vi "GetClassProperties.vi"(0 "reference in":refnum<class "ClassWriterGOOP400.lvclass">, 1 "LvClassItem":refnum<vi>, 2 "TreeControl":refnum<vi>, 5 "error in (no error)":errorcluster) -> (14 "reference out":refnum<class "ClassWriterGOOP400.lvclass">, 19 "error out":errorcluster)   [LabVIEW 2014, in "ClassWriterGOOP400.lvclass"]
uses:
  <resource>/Framework/Providers/Open_GDS/ClassProviders/Provider_EndevoGOOP400/ClassWriterGOOP400_class/ClassWriterGOOP400.lvclass
panel:
  out "ClassClasses":string[](array[string])
  out "ObjectClasses":string[](array[string])
  out "ClassAttributes":string[][](array[string])
  out "ObjectAttributes":string[][](array[string])
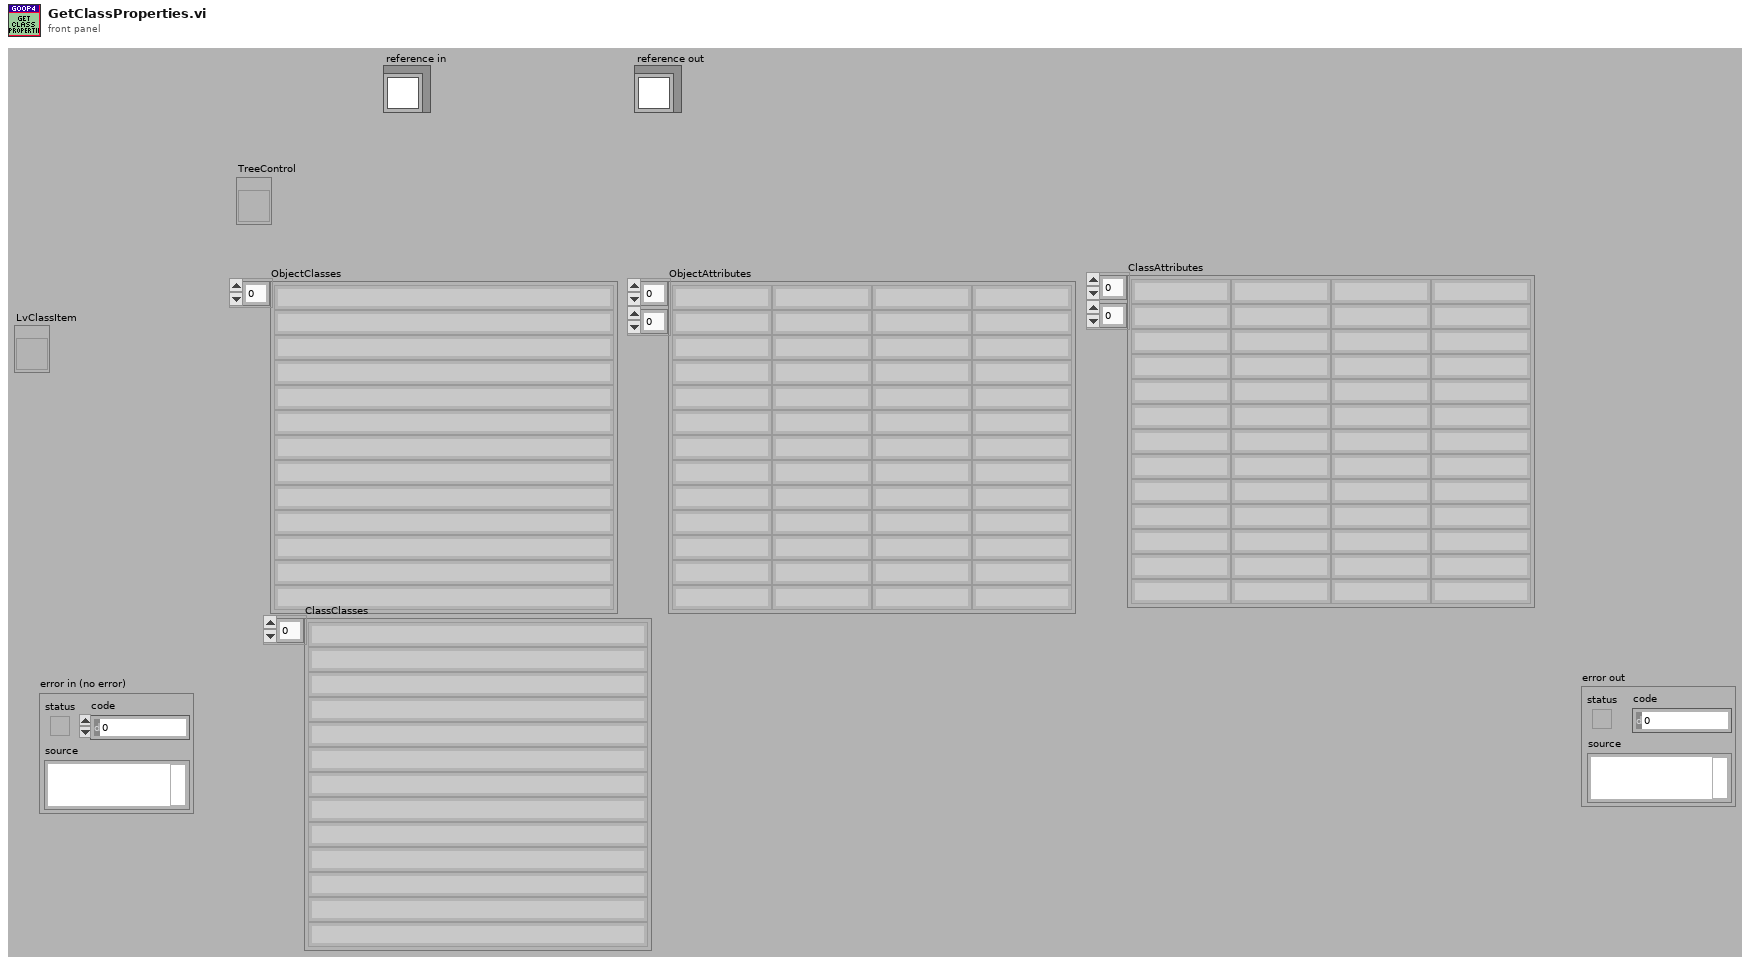
[diagram p1: front panel]
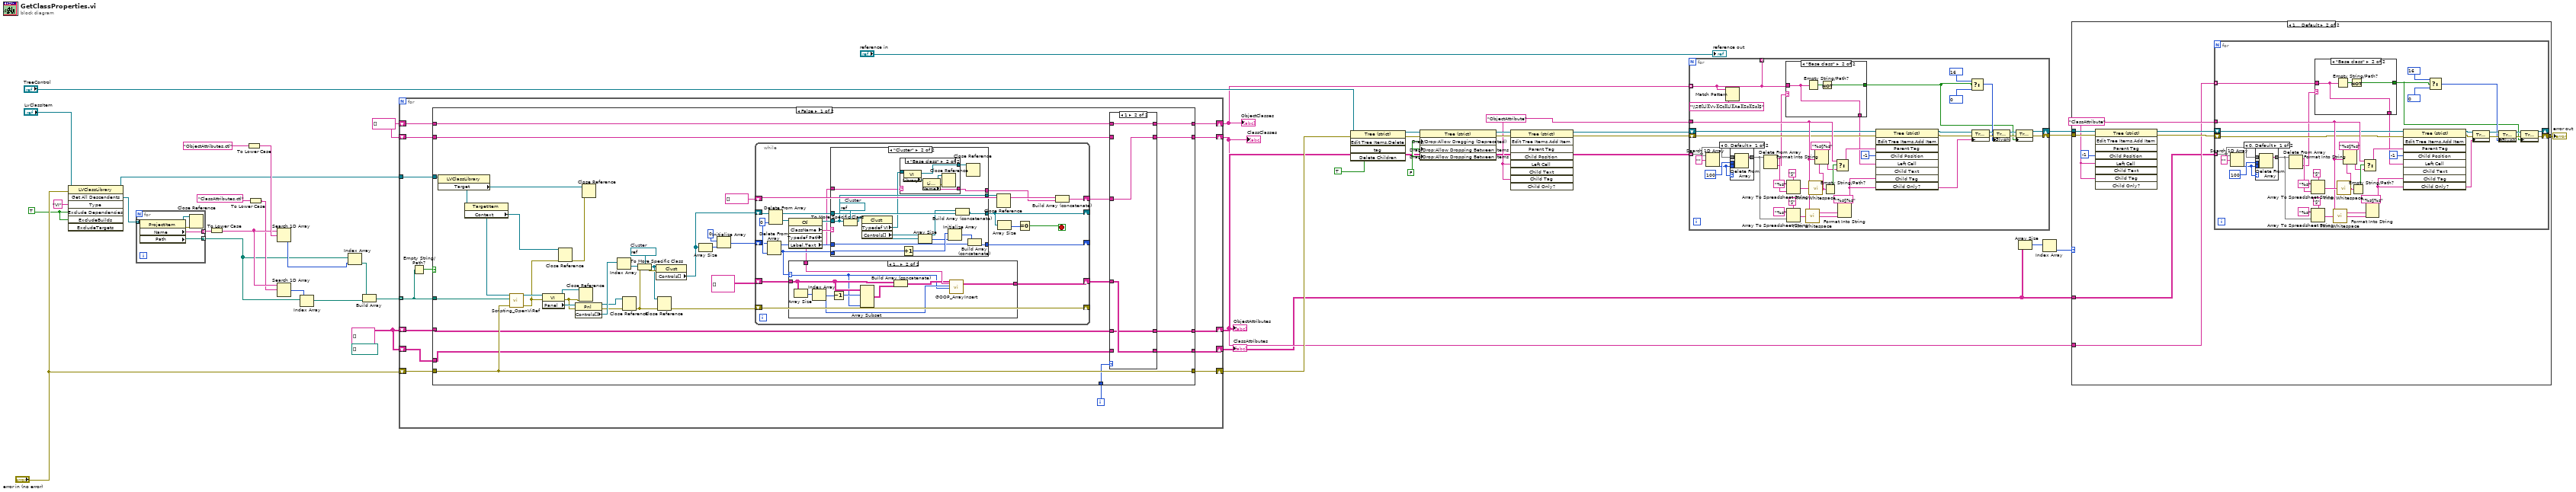
[diagram p0: block diagram]
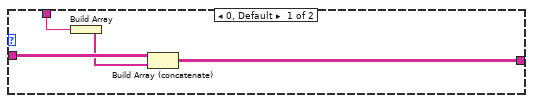
[diagram p8: hidden frame]
diagram:
  w5 = TRUE ("ExcludeDependencies")
  w17 = FALSE ("Drag/Drop:Allow Dragging (Deprecated)")
  w12 = "ObjectAttribute" ("Left Cell String(Main name)")
  w23 = string[] []
  (unwired) path[] []
  w40 = string[][] []
  n1 = invoke class="LVClassLibrary" method="Get All Descendents"(reference="LvClassItem", error in="error in (no error)", "Type"="VI", "Exclude Dependencies"=w5, "ExcludeBuilds"=w5) -> (reference out=w1:refnum<vi>, "All Descendents"=w38:refnum<vi>[])  [unwired: 2 in, 5 out]
  n2 = for {
    tunnel: w38 -> [w46] mode=indexing
    tunnel: [w45] -> w37 mode=indexing
    tunnel: [w44] -> w31 mode=indexing
    n3 = property class="ProjectItem"(reference=w46) -> (reference out=w43:refnum<vi>, error out=w42:errorcluster, "Name"=w45:string, "Path"=w44:path)  [unwired: 1 in]
    n4 = Close Reference(reference=w43, error in (no error)=w42) -> ()  [unwired: 1 out]
  }
  n5 = To Lower Case(string=w37) -> (all lower case string=w35:string[])
  n6 = To Lower Case(string="ObjectAttributes.ctl") -> (all lower case string=w36:string)
  n7 = To Lower Case(string="ClassAttributes.ctl") -> (all lower case string=w34:string)
  n8 = Search 1D Array(1D array=w35, element=w36) -> (index of element=w33:i32)  [unwired: 1 in]
  n9 = Search 1D Array(1D array=w35, element=w34) -> (index of element=w32:i32)  [unwired: 1 in]
  n10 = Index Array(array=w31, index=w32) -> (element=w25:path)
  n11 = Index Array(array=w31, index=w33) -> (element=w26:path)
  n12 = Build Array(w26, w25) -> (w30:path[])
  n13 = for {
    shift-right: [w60] -> w9
    shift-left: "error in (no error)" -> [w59]
    shift-right: [w57] -> w8
    shift-left: w40 -> [w58]
    shift-right: [w55] -> w4
    shift-left: w40 -> [w56]
    tunnel: w30 -> [w54] mode=indexing
    shift-right: [w51] -> w7
    shift-left: w23 -> [w48]
    shift-right: [w50] -> w6
    shift-left: w23 -> [w49]
    tunnel: w1 -> [w47]
    i -> [w52]
    n14 = Empty String/Path?(string/path=w54) -> (empty?=w53:bool)
    n15 = case shown="False" w53 {
      tunnel: [w95 w169] -> w60
      tunnel: w59 -> [w95 w169]
      tunnel: w58 -> [w79 w170]
      tunnel: [w82 w170] -> w57
      tunnel: w56 -> [w81 w168]
      tunnel: [w80 w168] -> w55
      tunnel: w54 -> [w97 _]
      tunnel: w52 -> [w84 _]
      tunnel: [w70 w167] -> w51
      tunnel: [w68 w166] -> w50
      tunnel: w49 -> [w67 w166]
      tunnel: w48 -> [w66 w167]
      tunnel: w47 -> [w64 _]
      frame False {
        w88 = refnum<vi> refnum  # Cluster
        n16 = property class="LVClassLibrary"(reference=w64) -> ("Target"=w65:refnum<vi>)  [unwired: 1 in, 2 out]
        n17 = property class="TargetItem"(reference=w65) -> ("Context"=w61:refnum<vi>)  [unwired: 1 in, 2 out]
        n18 = call <resource>:"Scripting_OpenViRef.vi"("error in"=w95, "ViPath/ViName/Viref"=w97, "AppRef"=w61) -> ("error out"=w63:errorcluster, "vi reference"=w96:refnum<vi>)  [unwired: 6 in, 1 out]
        n19 = property class="VI"(reference=w96, error in=w63) -> (reference out=w77:refnum<vi>, error out=w78:errorcluster, "Panel"=w94:refnum<vi>)
        n20 = Close Reference(reference=w61, error in (no error)=w63) -> (error out=w62:errorcluster)
        n21 = property class="Pnl"(reference=w94, error in=w78) -> (reference out=w72:refnum<vi>, error out=w74:errorcluster, "Controls[]"=w89:refnum<vi>[])
        n22 = Close Reference(reference=w77, error in (no error)=w78) -> ()  [unwired: 1 out]
        n23 = Close Reference(reference=w65, error in (no error)=w62) -> ()  [unwired: 1 out]
        n24 = Index Array(array=w89) -> (element=w87:refnum<vi>)  [unwired: 1 in]
        n25 = Close Reference(reference=w72, error in (no error)=w74) -> (error out=w73:errorcluster)
        n26 = To More Specific Class(target class=w88, reference=w87, error in=w73) -> (specific class reference=w76:refnum<vi>, error out=w86:errorcluster)
        n27 = property class="Clust"(reference=w76, error in=w86) -> ("Controls[]"=w85:refnum<vi>[])  [unwired: 2 out]
        n28 = Close Reference(reference=w76, error in (no error)=w73) -> (error out=w75:errorcluster)
        n29 = Array Size(array=w85) -> (size(s)=w92:i32)
        n30 = Initialize Array(0 ("index"), w92) -> (w90:i32[])
        n31 = while {
          shift-right: [w124] -> _
          shift-left: w85 -> [w126]
          shift-right: [w111] -> _
          shift-left: w75 -> [w111]
          shift-right: [w119] -> w83
          shift-left: string[][] [] -> [w120]
          shift-right: [w113] -> _
          shift-left: w90 -> [w115]
          shift-right: [w108] -> w69
          shift-left: string[] [] -> [w109]
          stop <- w122 stop-if-true
          w116 = 0 ("index")
          n32 = Delete From Array(array=w115, index=w116) -> (deleted portion=w112:i32, array with subset deleted=w114:i32[])  [unwired: 1 in]
          n33 = Delete From Array(array=w126, index=w116) -> (deleted portion=w121:refnum<vi>, array with subset deleted=w125:refnum<vi>[])  [unwired: 1 in]
          n34 = property class="Ctl" props=["ClassName", "Typedef Path", "Label", "Text"](reference=w121) -> (reference out=w117:refnum<vi>, "ClassName"=w118:string, "Label.Text"=w106:string)  [unwired: 1 in, 2 out]
          n35 = case shown="1.." w112 {
            selector: w112 -> [_ w131]
            tunnel: w120 -> [w130 w135]
            tunnel: [w129 w138] -> w119
            tunnel: w106 -> [w128 w137]
            frame 0, Default {
              n36 = Build Array(w128) -> (w127:string[])
              n37 = Build Array (concatenate)(w130, w127) -> (w129:string[][])
            }
            frame 1.. {
              n38 = Array Size(array=w135) -> (size(s)=w139:i32[])
              n39 = Index Array(array=w139) -> (element=w133:i32)  [unwired: 1 in]
              n40 = Decrement(x=w133) -> (x-1=w132:i32)
              n41 = Array Subset(array=w135, index (row)=w132, length (col)=w131) -> (w134:string[][])  [unwired: 2 in]
              n42 = Build Array (concatenate)(w135, w134) -> (w136:string[][])
              n43 = call <resource>:"GOOP_ArrayInsert.vi"("ArrayIn"=w136, "Text"=w137, "Row"=w133, "Column"=w131) -> ("ArrayOut"=w138:string[][])  [unwired: 15 in]
            }
          }
          n44 = case shown="\"Cluster\"" w118 {
            tunnel: [w142 w156] -> w124
            tunnel: w125 -> [w142 w155]
            tunnel: w117 -> [w140 w147]
            tunnel: w114 -> [w141 w149]
            tunnel: [w141 w150] -> w113
            tunnel: w112 -> [_ w153]
            tunnel: [w140 w147] -> w110
            tunnel: [_ w145] -> w107
            tunnel: w106 -> [_ w143]
            frame Default {
            }
            frame "Cluster" {
              w158 = refnum<vi> refnum  # Cluster
              n45 = To More Specific Class(target class=w158, reference=w147) -> (specific class reference=w157:refnum<vi>)  [unwired: 1 in, 1 out]
              n46 = property class="Clust"(reference=w157) -> ("Typedef VI"=w146:refnum<vi>, "Controls[]"=w154:refnum<vi>[])  [unwired: 1 in, 2 out]
              n47 = case shown="\"Base class\"" w143 {
                tunnel: w146 -> [w159 w165]
                tunnel: [_ w163] -> w145
                tunnel: [w159 w160] -> w144
                frame "False", Default {
                }
                frame "Base class" {
                  n48 = property class="VI"(reference=w165) -> (reference out=w160:refnum<vi>, "Library"=w164:refnum<vi>)  [unwired: 1 in, 1 out]
                  n49 = property class="Library"(reference=w164) -> (reference out=w162:refnum<vi>, error out=w161:errorcluster, "Name"=w163:string)  [unwired: 1 in]
                  n50 = Close Reference(reference=w162, error in (no error)=w161) -> ()  [unwired: 1 out]
                }
              }
              n51 = Increment(x=w153) -> (x+1=w152:i32)
              n52 = Array Size(array=w154) -> (size(s)=w151:i32)
              n53 = Initialize Array(w152, w151) -> (w148:i32[])
              n54 = Build Array (concatenate)(w154, w155) -> (w156:refnum<vi>[])
              n55 = Close Reference(reference=w144) -> ()  [unwired: 1 in, 1 out]
              n56 = Build Array (concatenate)(w148, w149) -> (w150:i32[])
            }
          }
          n57 = Close Reference(reference=w110) -> ()  [unwired: 1 in, 1 out]
          n58 = Array Size(array=w124) -> (size(s)=w123:i32)
          n59 = Equal To 0?(x=w123) -> (x = 0?=w122:bool)
          n60 = Build Array (concatenate)(w109, w107) -> (w108:string[])
        }
        n61 = case shown="1" w84 {
          tunnel: [w101 w104] -> w82
          tunnel: w83 -> [w101 w105]
          tunnel: w81 -> [w100 _]
          tunnel: [w100 w105] -> w80
          tunnel: w79 -> [_ w104]
          tunnel: [w99 w103] -> w70
          tunnel: w69 -> [w99 w102]
          tunnel: [w98 w102] -> w68
          tunnel: w67 -> [w98 _]
          tunnel: w66 -> [_ w103]
          frame 0, Default {
          }
          frame 1 {
          }
        }
      }
      frame True {
      }
    }
  }
  "ObjectAttributes" <- w8
  "ClassAttributes" <- w4
  "ObjectClasses" <- w7
  "ClassClasses" <- w6
  n62 = invoke on="Invoke Node" class="Tree (strict)" method="Edit Tree Items.Delete"(reference="TreeControl", error in=w9, "Delete Children"=TRUE) -> (reference out=w21:refnum<vi>, error out=w20:errorcluster)  [unwired: 2 in, 3 out]
  n63 = property class="Tree (strict)"(reference=w21, error in=w20, "Drag/Drop:Allow Dragging (Deprecated)"=w17, "Drag/Drop:Allow Dropping Between Items"=w17, "Drag/Drop:Allow Dropping Between Items"=w17) -> (reference out=w19:refnum<vi>, error out=w18:errorcluster)
  n64 = invoke on="Invoke Node" class="Tree (strict)" method="Edit Tree Items.Add Item"(reference=w19, error in=w18, "Left Cell"=w12, "Child Tag"=w12) -> (reference out=w11:refnum<vi>, error out=w10:errorcluster)  [unwired: 5 in, 7 out]
  n65 = for {
    shift-right: [w173] -> w15
    shift-left: w10 -> [w190]
    shift-right: [w172] -> w16
    shift-left: w11 -> [w189]
    tunnel: w8 -> [w209] mode=indexing
    tunnel: w12 -> [w192]
    tunnel: w7 -> [w179] mode=indexing
    tunnel: [w179] -> _ mode=indexing
    n66 = Search 1D Array(1D array=w209, element="") -> (index of element=w198:i32)  [unwired: 1 in]
    n67 = Match Pattern(string=w179, regular expression="\\2E[Ll][Vv][Cc][Ll][Aa][Ss][Ss]$") -> ()  [unwired: 1 in, 4 out]
    n68 = case shown="0, Default" w198 {
      tunnel: w198 -> [w218 _]
      tunnel: w209 -> [w217 w219]
      tunnel: 100 ("length") -> [w216 _]
      tunnel: [w215 w219] -> w199
      frame 0, Default {
        n69 = Delete From Array(array=w217, length=w216, index=w218) -> (array with subset deleted=w215:string[])  [unwired: 1 out]
      }
      frame -1 {
      }
    }
    n70 = Delete From Array(array=w199) -> (deleted portion=w187:string, array with subset deleted=w207:string[])  [unwired: 2 in]
    n71 = case shown="\"Base class\"" w187 {
      selector: w187 -> [w211 _]
      tunnel: [w211 w212] -> w186
      tunnel: w179 -> [_ w212]
      tunnel: [_ w213] -> w171
      frame Default {
      }
      frame "Base class" {
        n72 = Empty String/Path?(string/path=w212) -> (empty?=w214:bool)
        n73 = Not(x=w214) -> (.not. x?=w213:bool)
      }
    }
    n74 = Array To Spreadsheet String(delimiter (Tab)="§", array=w207, 3:"%s" ("format string")) -> (spreadsheet string=w204:string)
    n75 = Array To Spreadsheet String(delimiter (Tab)="§", array=w199, 3:"%s" ("format string")) -> (spreadsheet string=w202:string)
    n76 = call <vilib>:"Trim Whitespace.vi"("string"=w202) -> ("trimmed string"=w193:string)  [unwired: 1 in]
    n77 = call <vilib>:"Trim Whitespace.vi"("string"=w204) -> ("trimmed string"=w196:string)  [unwired: 1 in]
    n78 = Format Into String(format string="%s§%s", w192, w196) -> (resulting string=w195:string)  [unwired: 2 in, 1 out]
    n79 = Empty String/Path?(string/path=w196) -> (empty?=w203:bool)
    n80 = Select(t=w192, s=w203, f=w195) -> (s? t:f=w191:string)
    n81 = Format Into String(format string="%s§%s", w192, w193) -> (resulting string=w180:string)  [unwired: 2 in, 1 out]
    n82 = invoke on="Invoke Node" class="Tree (strict)" method="Edit Tree Items.Add Item"(reference=w189, error in=w190, "Parent Tag"=w191, "Child Position"=-1, "Left Cell"=w186, "Child Tag"=w180) -> (reference out=w182:refnum<vi>, error out=w181:errorcluster)  [unwired: 3 in, 7 out]
    n83 = Select(t=16, s=w171, f=0) -> (s? t:f=w176:i32)
    n84 = property class="Tree (strict)"(reference=w182, error in=w181, "Active Item Tag"=w180) -> (reference out=w184:refnum<vi>, error out=w183:errorcluster)
    n85 = property class="Tree (strict)"(reference=w184, error in=w183, "Glyph"=w176) -> (reference out=w175:refnum<vi>, error out=w174:errorcluster)
    n86 = property class="Tree (strict)"(reference=w175, error in=w174, "Disabled?"=w171) -> (reference out=w172:refnum<vi>, error out=w173:errorcluster)
  }
  n87 = Array Size(array=w4) -> (size(s)=w3:i32[])
  n88 = Index Array(array=w3) -> (element=w2:i32)  [unwired: 1 in]
  n89 = case shown="1.., Default" w2 {
    tunnel: w16 -> [_ w229]
    tunnel: w15 -> [w220 w228]
    tunnel: [w220 w227] -> w14
    tunnel: w6 -> [_ w222]
    tunnel: w4 -> [_ w221]
    frame 0 {
    }
    frame 1.., Default {
      w225 = "ClassAttribute" ("Left Cell String(Main name)")
      n90 = invoke on="Invoke Node" class="Tree (strict)" method="Edit Tree Items.Add Item"(reference=w229, error in=w228, "Child Position"=-1, "Left Cell"=w225, "Child Tag"=w225) -> (reference out=w224:refnum<vi>, error out=w223:errorcluster)  [unwired: 4 in, 7 out]
      n91 = for {
        shift-right: [w232] -> w227
        shift-left: w223 -> [w248]
        shift-right: [w231] -> _
        shift-left: w224 -> [w247]
        tunnel: w221 -> [w267] mode=indexing
        tunnel: w225 -> [w250]
        tunnel: w222 -> [w238] mode=indexing
        n92 = Search 1D Array(1D array=w267, element="") -> (index of element=w256:i32)  [unwired: 1 in]
        n93 = case shown="0, Default" w256 {
          tunnel: w256 -> [w276 _]
          tunnel: w267 -> [w275 w277]
          tunnel: 100 ("length") -> [w274 _]
          tunnel: [w273 w277] -> w257
          frame 0, Default {
            n94 = Delete From Array(array=w275, length=w274, index=w276) -> (array with subset deleted=w273:string[])  [unwired: 1 out]
          }
          frame -1 {
          }
        }
        n95 = Delete From Array(array=w257) -> (deleted portion=w245:string, array with subset deleted=w265:string[])  [unwired: 2 in]
        n96 = Array To Spreadsheet String(delimiter (Tab)="§", array=w265, 3:"%s" ("format string")) -> (spreadsheet string=w262:string)
        n97 = Array To Spreadsheet String(delimiter (Tab)="§", array=w257, 3:"%s" ("format string")) -> (spreadsheet string=w260:string)
        n98 = case shown="\"Base class\"" w245 {
          selector: w245 -> [w269 _]
          tunnel: [w269 w270] -> w244
          tunnel: w238 -> [_ w270]
          tunnel: [_ w271] -> w230
          frame Default {
          }
          frame "Base class" {
            n99 = Empty String/Path?(string/path=w270) -> (empty?=w272:bool)
            n100 = Not(x=w272) -> (.not. x?=w271:bool)
          }
        }
        n101 = call <vilib>:"Trim Whitespace.vi"("string"=w260) -> ("trimmed string"=w251:string)  [unwired: 1 in]
        n102 = call <vilib>:"Trim Whitespace.vi"("string"=w262) -> ("trimmed string"=w254:string)  [unwired: 1 in]
        n103 = Format Into String(format string="%s§%s", w250, w254) -> (resulting string=w253:string)  [unwired: 2 in, 1 out]
        n104 = Empty String/Path?(string/path=w254) -> (empty?=w261:bool)
        n105 = Select(t=w250, s=w261, f=w253) -> (s? t:f=w249:string)
        n106 = Format Into String(format string="%s§%s", w250, w251) -> (resulting string=w239:string)  [unwired: 2 in, 1 out]
        n107 = invoke on="Invoke Node" class="Tree (strict)" method="Edit Tree Items.Add Item"(reference=w247, error in=w248, "Parent Tag"=w249, "Child Position"=-1, "Left Cell"=w244, "Child Tag"=w239) -> (reference out=w241:refnum<vi>, error out=w240:errorcluster)  [unwired: 3 in, 7 out]
        n108 = Select(t=16, s=w230, f=0) -> (s? t:f=w236:i32)
        n109 = property class="Tree (strict)"(reference=w241, error in=w240, "Active Item Tag"=w239) -> (reference out=w243:refnum<vi>, error out=w242:errorcluster)
        n110 = property class="Tree (strict)"(reference=w243, error in=w242, "Glyph"=w236) -> (reference out=w234:refnum<vi>, error out=w233:errorcluster)
        n111 = property class="Tree (strict)"(reference=w234, error in=w233, "Disabled?"=w230) -> (reference out=w231:refnum<vi>, error out=w232:errorcluster)
      }
    }
  }
  "error out" <- w14
  "reference out" <- "reference in"
